vi "Split Type and Data from JSON.vi"(10 "<JSON>":string) -> (1 "Data":string, 2 "Type":string)   [LabVIEW 2017, in "JSON Serializable Serializer.lvclass"]
doc: "Splits <B>Type</B> and <B>Data</B> from JSON. The type name is expected to be in the \"$type\" field and data is either in a \"$data\" field or whatever remains after removing the \"$type\" field."
uses:
  JSON Serializable Serializer.lvclass
  <vilib>/JDP Science/JSONtext/JSONtext.lvlib
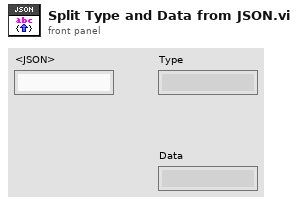
[diagram p1: front panel]
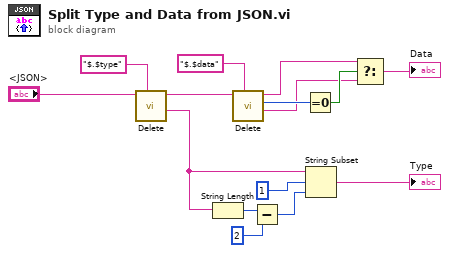
[diagram p0: block diagram]
diagram:
  n1 = call <vilib>:"Delete.vi"("$Path or Item Name"="$.$type", "JSON"="<JSON>") -> ("<JSON> First Deleted Item"=w4:string, "<JSON>"=w12:string)  [unwired: 5 in, 2 out]
  n2 = String Length(string=w4) -> (length=w3:i32)
  n3 = call <vilib>:"Delete.vi"("$Path or Item Name"="$.$data", "JSON"=w12) -> ("<JSON> First Deleted Item"=w8:string, "Number Deleted"=w11:i32, "<JSON>"=w9:string)  [unwired: 5 in, 1 out]
  n4 = Subtract(x=w3, y=2) -> (x-y=w1:i32)
  n5 = Equal To 0?(x=w11) -> (x = 0?=w10:bool)
  n6 = String Subset(string=w4, offset (0)=1, length (rest)=w1) -> (substring=→"Type":string)
  n7 = Select(t=w9, s=w10, f=w8) -> (s? t:f=→"Data":string)
